vi "Read object names.vi"(10 "Error In":errorcluster, 11 "Menu object array ref":refnum<vi>) -> (2 "Error Out":errorcluster, 3 "Object names":string[](array[string]))   [LabVIEW 2015]
uses:
  Controls/Menu object.ctl
panel:
  in  "Object name":u16(ring) items=["Select one"]
  in  "Menu object":T1 {"Object name" items=["Select one"]}
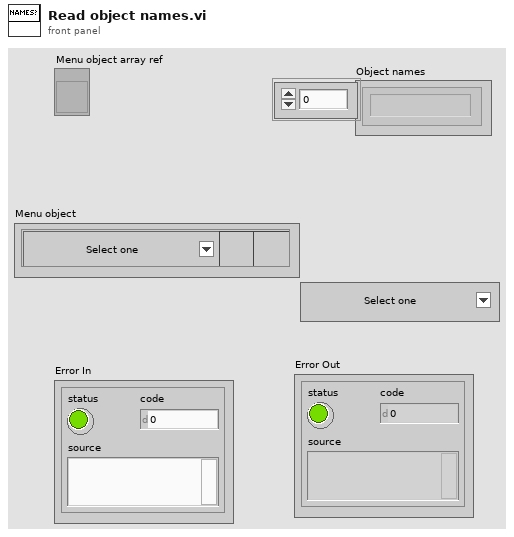
[diagram p1: front panel]
types:
  T1 = typedef "Menu object.ctl" = cluster{"Object name":u16, "Open parameters":bool, "Remove Button":bool}
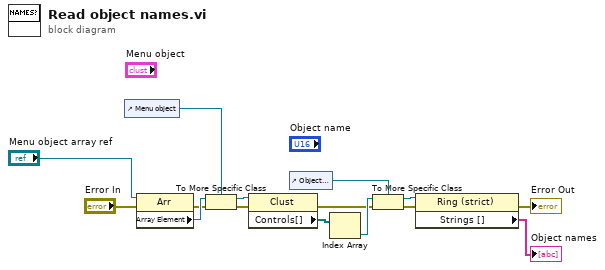
[diagram p0: block diagram]
diagram:
  n1 = control-ref of="Menu object"() -> (w14:refnum<vi>)
  n2 = property class="Arr"(reference="Menu object array ref", error in="Error In") -> (error out=w5:errorcluster, "Array Element"=w15:refnum<vi>)  [unwired: 1 out]
  n3 = To More Specific Class(target class=w14, reference=w15, error in=w5) -> (specific class reference=w13:refnum<vi>, error out=w4:errorcluster)
  n4 = property class="Clust"(reference=w13, error in=w4) -> (error out=w3:errorcluster, "Controls[]"=w9:refnum<vi>[])  [unwired: 1 out]
  n5 = control-ref of="Object name"() -> (w12:refnum<vi>)
  n6 = Index Array(array=w9) -> (element=w10:refnum<vi>)  [unwired: 1 in]
  n7 = To More Specific Class(target class=w12, reference=w10, error in=w3) -> (specific class reference=w11:refnum<vi>, error out=w2:errorcluster)
  n8 = property class="Ring (strict)"(reference=w11, error in=w2) -> (error out=→"Error Out":errorcluster, "Strings []"=→"Object names":string[])  [unwired: 1 out]
